vi "Audio Data Format To ma_format.vi"(11 "Format":T1) -> (3 "ma_format":u16)   [LabVIEW 2020, in "G-Audio.lvlib"]
uses:
  G-Audio.lvlib
  Controls/Audio Device Format.ctl
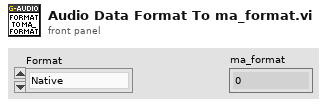
[diagram p1: front panel]
types:
  T1 = typedef "G-Audio.lvlib/Audio Device Format.ctl" = enum16{"Native", "U8", "I16", "I32", "F32"}
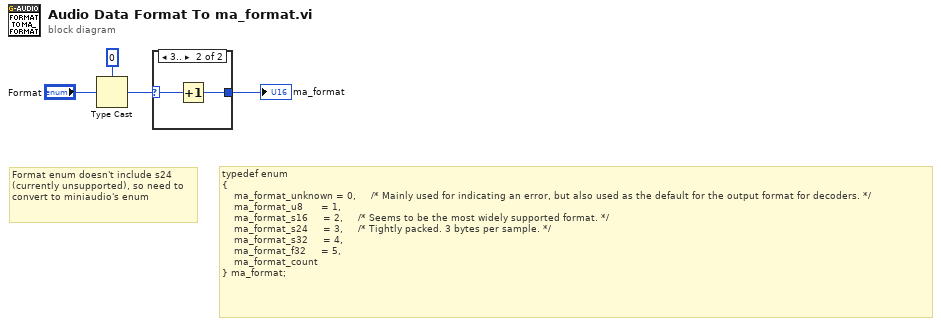
[diagram p0: block diagram]
diagram:
  # "Format enum doesn't include s24 (currently unsupported), so need to convert to miniaudio's enum"
  # "typedef enum\n{\n    ma_format_unknown = 0,     /* Mainly used for indicating an error, but also used as the default for the output format for decoders. */\n    ma_format_u8      = 1,\n    ma_format_s16     = 2,     /* Seems to be the most widely supported format. */\n    ma_format_s24     = 3,     /* Tightly packed. 3 bytes per sample. */\n    ma_format_s32     = 4,\n    ma_format_f32     = 5,\n    ma_format_count\n} ma_format;"
  n1 = Type Cast(type=u16 0, x="Format") -> (*(type *) &x=w1:u16)
  n2 = case shown="3.." w1 {
    selector: w1 -> [w5 w7]
    tunnel: [w5 w6] -> w4
    frame Default {
    }
    frame 3.. {
      n3 = Increment(x=w7) -> (x+1=w6:u16)
    }
  }
  "ma_format" <- w4
